vi "PL_Scan.vi"() -> ()   [LabVIEW 2020]
uses:
  PL_Global.vi
panel:
  out "Resulting String":string
  in  "STOP":bool
  in  "Name":string
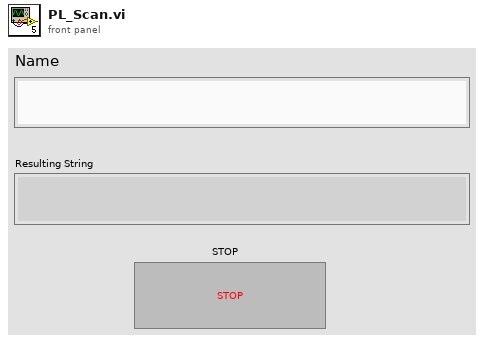
[diagram p1: front panel]
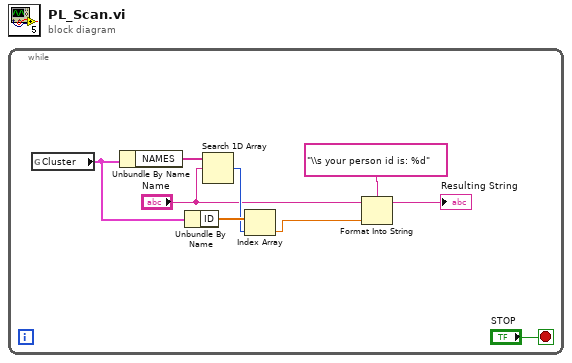
[diagram p0: block diagram]
diagram:
  n1 = while {
    stop <- "STOP" stop-if-true
    n2 = global read "PL_Global.vi" "Cluster"() -> (w7:cluster{"NAMES":string[], "ID":dbl[]})
    n3 = Unbundle By Name(w7) -> ("NAMES"=w8:string[])
    n4 = Unbundle By Name(w7) -> ("ID"=w6:dbl[])
    n5 = Search 1D Array(1D array=w8, element="Name") -> (index of element=w5:i32)  [unwired: 1 in]
    n6 = Index Array(array=w6, index=w5) -> (element=w2:dbl)
    n7 = Format Into String(format string="\\s your person id is: %d", initial string="Name", w2) -> (resulting string=→"Resulting String":string)  [unwired: 1 in, 1 out]
  }
